vi "Draw.vi"(7 "menu in":refnum<class "menu.lvclass">, 8 "error in (no error)":errorcluster, 11 "arrow in":refnum<class "arrow.lvclass">) -> (0 "error out":errorcluster, 3 "arrow out":refnum<class "arrow.lvclass">)   [LabVIEW 2009, in "arrow.lvclass"]
uses:
  arrow.lvclass
  Menu/menu.lvclass
  arrow.lvclass/arrow.ctl
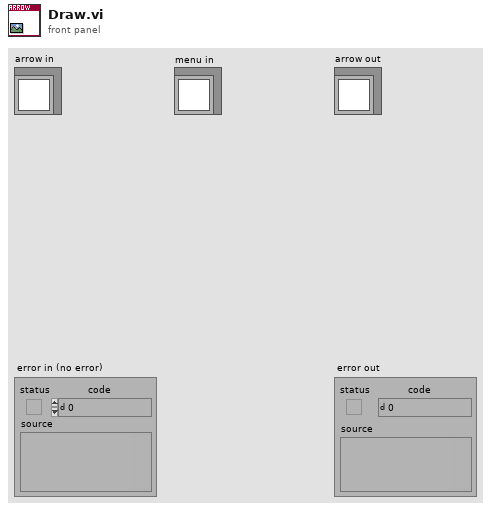
[diagram p1: front panel]
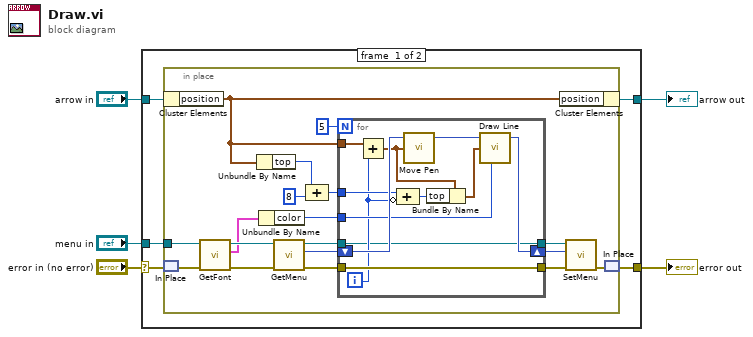
[diagram p0: block diagram]
diagram:
  n1 = case shown="No Error" "error in (no error)" {
    selector: "error in (no error)" -> [w7 w42]
    tunnel: [w6 w42] -> w2
    tunnel: [w9 w41] -> w4
    tunnel: "arrow in" -> [w10 w41]
    tunnel: "menu in" -> [w8 _]
    frame #0 {
      n2 = in-place {
        in-place-border: w8 -> [w28]
        n3 = in-place-cluster #1(w10) -> ("position"=w14:cluster{"left":u32, "top":u32})
        n4 = in-place-match #2(w7) -> (w27:errorcluster)
        n5 = call "GetFont.vi"("error in (no error)"=w27, "menu in"=w28) -> ("error out"=w26:errorcluster, "font"=w17:cluster{"name":string, "size":i16, "color":u32}, "menu out"=w25:refnum<class "menu.lvclass">)  [unwired: 7 in]
        n6 = Unbundle By Name(w14) -> ("top"=w12:u32)
        n7 = Unbundle By Name(w17) -> ("color"=w16:u32)
        n8 = call "GetMenu.vi"("error in (no error)"=w26, "menu in"=w25) -> ("error out"=w22:errorcluster, "menu"=w23:picture, "menu out"=w24:refnum<class "menu.lvclass">)  [unwired: 7 in]
        n9 = Compound Arithmetic op=ADD(w12, u32 8 ("value")) -> (w13:u32)
        n10 = for {
          N: 5 -> [_]
          shift-right: [w37] -> w18
          shift-left: w23 -> [w40]
          tunnel: w14 -> [w39]
          tunnel: w16 -> [w36]
          tunnel: w13 -> [w33]
          tunnel: w22 -> [w35]
          tunnel: [w35] -> w21
          tunnel: w24 -> [w30]
          tunnel: [w30] -> w19
          i -> [w31]
          n11 = Add(x=w39, y=w31) -> (x+y=w34:cluster{"left":u32, "top":u32})
          n12 = Compound Arithmetic op=ADD(w33, invert w31) -> (w32:u32)
          n13 = call <vilib>:"Move Pen.vi"("new position"=w34, "picture"=w40) -> ("new picture"=w38:picture)  [unwired: 3 in]
          n14 = Bundle By Name(cluster=w34, "top"=w32) -> (w29:cluster{"left":u32, "top":u32})
          n15 = call <vilib>:"Draw Line.vi"("picture"=w38, "end point"=w29, "color(black)"=w36) -> ("new picture"=w37:picture)  [unwired: 6 in]
        }
        n16 = in-place-cluster #1("position"=w14) -> (w9:refnum<class "arrow.lvclass">)
        n17 = call "SetMenu.vi"("error in (no error)"=w21, "menu"=w18, "menu in"=w19) -> ("error out"=w20:errorcluster)  [unwired: 7 in, 1 out]
        n18 = in-place-match #2(w20) -> (w6:errorcluster)
      }
    }
    frame #1 {
    }
  }
  "arrow out" <- w4
  "error out" <- w2
